vi "Trim Whitespace and Separator.vi"(11 "Measurement value":string) -> (3 "trimmed string":string)   [LabVIEW 2021]
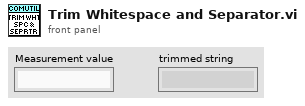
[diagram p1: front panel]
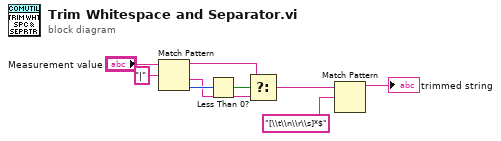
[diagram p0: block diagram]
diagram:
  n1 = Match Pattern(string="Measurement value", regular expression="|") -> (before substring=w5:string, after substring=w4:string, offset past match=w7:i32)  [unwired: 1 in, 1 out]
  n2 = Less Than 0?(x=w7) -> (x < 0?=w6:bool)
  n3 = Select(t=w5, s=w6, f=w4) -> (s? t:f=w3:string)
  n4 = Match Pattern(string=w3, regular expression="[\\t\\n\\r\\s]*$") -> (before substring=→"trimmed string":string)  [unwired: 1 in, 3 out]
